vi "Read Key String.vi"(6 "Default Val":string, 7 "Section Name":string, 8 "error in (no error)":errorcluster, 10 "Key Names":string, 11 "Config Data":T1(array[cluster])) -> (0 "error out":errorcluster, 1 "Key Names":string[](array[string]), 2 "Key Val out":string, 3 "Config Data dup":T1(array[cluster]), 4 "Key Find?":bool)   [LabVIEW 2020, in "GUCalibration2.lvlib"]
uses:
  GUCalibration2.lvlib
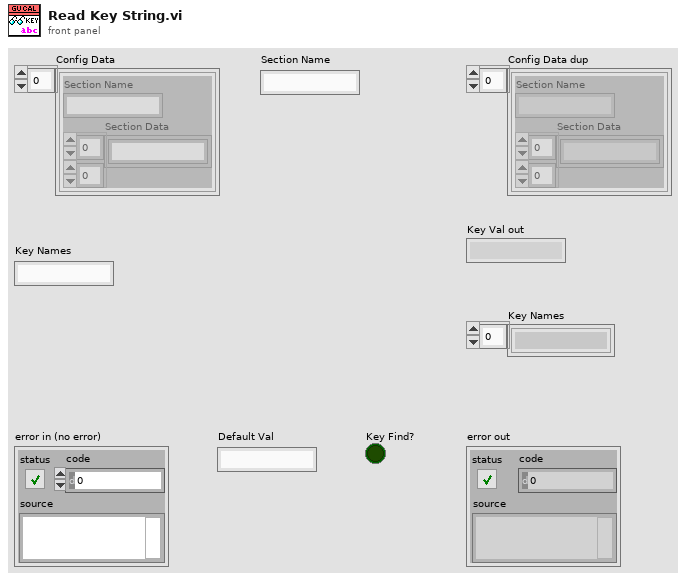
[diagram p1: front panel]
types:
  T1 = cluster{"Section Name":string, "Section Data":string[][]}[]
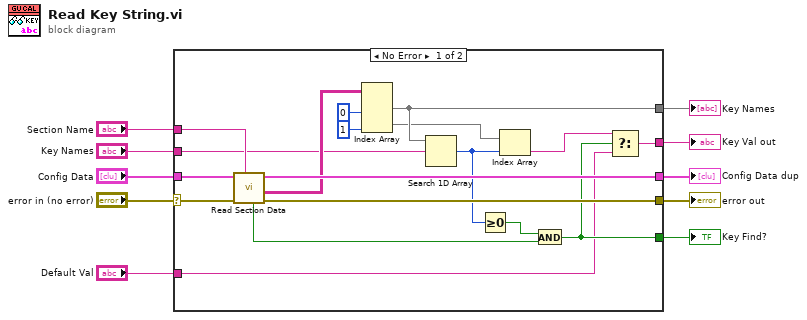
[diagram p0: block diagram]
diagram:
  n1 = case shown="No Error" "error in (no error)" {
    selector: "error in (no error)" -> [w26 w30]
    tunnel: "Section Name" -> [w27 _]
    tunnel: "Config Data" -> [w28 w29]
    tunnel: [w20 w30] -> w7
    tunnel: [w25 w29] -> w6
    tunnel: [w22 _] -> w5
    tunnel: "Key Names" -> [w21 _]
    tunnel: [w11 _] -> w3
    tunnel: [w14 _] -> w2
    tunnel: "Default Val" -> [w12 _]
    frame No Error {
      n2 = call "Read Section Data.vi"("Section Name"=w27, "error in (no error)"=w26, "Config Data"=w28) -> ("error out"=w20:errorcluster, "Section Data"=w24:string[][], "Config Data out"=w25:T1, "Section Exist"=w15:bool)  [unwired: 4 in, 1 out]
      n3 = Index Array(array=w24, index (col) #1=0 ("disabled index (col)"), index (col) #2=1 ("index (col)")) -> (element #1=w22:string[], element #2=w18:string[])  [unwired: 2 in]
      n4 = Search 1D Array(1D array=w22, element=w21) -> (index of element=w17:i32)  [unwired: 1 in]
      n5 = Greater Or Equal To 0?(x=w17) -> (x >= 0?=w16:bool)
      n6 = Index Array(array=w18, index=w17) -> (element=w13:string)
      n7 = And(x=w16, y=w15) -> (x .and. y?=w14:bool)
      n8 = Select(t=w13, s=w14, f=w12) -> (s? t:f=w11:string)
    }
    frame Error {
    }
  }
  "error out" <- w7
  "Key Names" <- w5
  "Config Data dup" <- w6
  "Key Val out" <- w3
  "Key Find?" <- w2
